vi "Process.vi"(0 "reference in":refnum<class "Battery.lvclass">, 5 "error in":errorcluster) -> (14 "reference out":refnum<class "Battery.lvclass">, 19 "error out":errorcluster)   [LabVIEW 2023, in "Battery.lvclass"]
uses:
  Battery.lvclass
  Model Parameters.ctl
  Simulation Parameters.ctl
  builds/PowerModuleInterface/PowerModuleInterface.lvlibp/Classes/PowerModule_interface/PowerModuleInterface.lvclass
  Battery.lvclass/Battery.ctl
  <vilib>/Utility/SystemLogging/NI_SystemLogging.lvlib
  <userlib>/_OpenG.lib/time/time.llb/openg_time.lvlib
panel:
  out "error info":errorcluster
  in  "Battery Tab Control":enum32{"MODEL", "SIMULATION", "PARAM"}(tab)
  out "SOC OCV Curve":cluster{"[0]":dbl, "[1]":dbl}[](graph)
  out "State of Charge %":dbl(slide)=100.0 caption="State of Charge (%)" scale=0.0..100.0 scale format="%.2g"
  out "Terminal Voltage (V)":dbl format="%#.3g"
  out "Battery Simulation":dbl[][](graph)
  out "Running Status Log":i32(listbox) caption="TEST SERVER LOG"
  out "Temperature (C)":dbl=25.0 format="%.2g"
  in  "Simulation Parameters":T1={"num_rc_pairs"=1, "R0"=0.0015, "R1"=0.001, "C1"=2500.0, "R2"=0.0008, "C2"=40000.0, " nominal_capacity_Ah"=5.0, "upper_voltage_cutoff"=4.2, "lower_voltage_cutoff"=3.0} {"lower_voltage_cutoff" format="%#_13g"; "upper_voltage_cutoff" format="%#_13g"; "nominal_capacity_Ah" format="%#_13g"; "C2" format="%#_13g"; "R2" format="%#_13g"; "C1" format="%#_13g"; "R1" format="%#_13g"; "R0" format="%#_13g"}
  in  "Model Parameters":T2={"chemistry"="Chen2020", "model_type"="SPMe"}
  out "Last Command":string
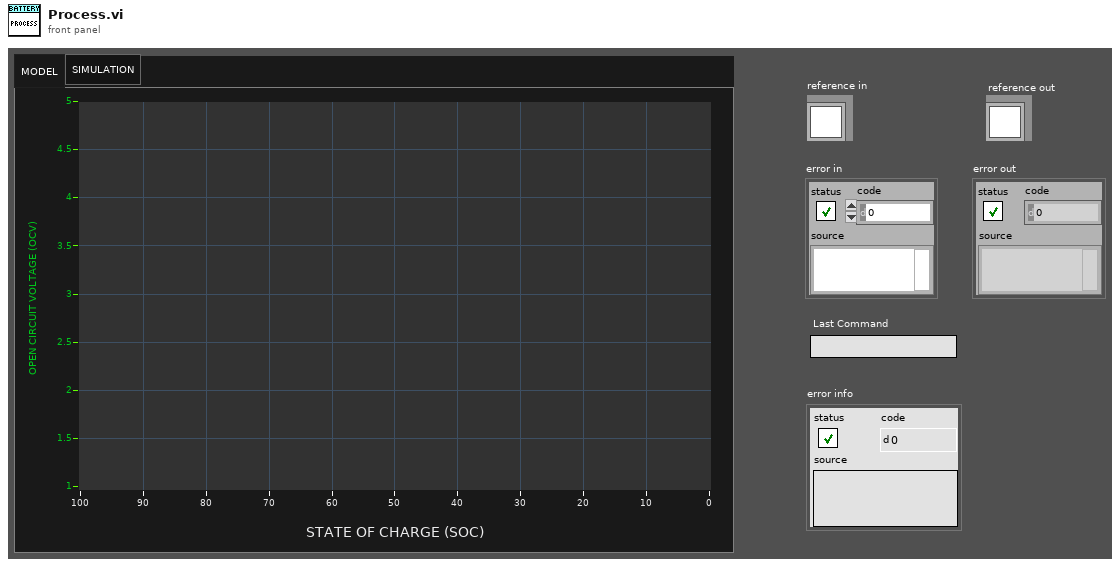
[diagram p1: front panel]
types:
  T1 = typedef "Battery.lvclass/Simulation Parameters.ctl" = cluster{"num_rc_pairs":i32, "R0":dbl, "R1":dbl, "C1":dbl, "R2":dbl, "C2":dbl, " nominal_capacity_Ah":dbl, "upper_voltage_cutoff":dbl, "lower_voltage_cutoff":dbl}
  T2 = typedef "Battery.lvclass/Model Parameters.ctl" = cluster{"chemistry":string, "model_type":string}
  T3 = cluster{"Core":cluster{"Timeout":i32, "Events":cluster{"EventsToProcess":refnum<event-registration>}, "EventFromProcess":refnum<user-event>, "ProcessSyncQueue":refnum<queue>, "QueueFromProcess":refnum<queue>, "Command":string, "Data":variant}}
  T4 = enum32{"Invalid", "Standard", "Closed", "Hidden", "Minimized", "Maximized"}
  T5 = cluster{"EventsToProcess":refnum<event-registration>}
  T6 = typedef "Battery.lvclass/ObjectAttributes.ctl" = cluster{"Python module":path, "Python Session":refnum<k35>, "PybammWrapper":refnum<k38>, "model loaded":bool, "simulation loaded":bool, "simulation enabled":bool, "SOC OCV Curve":dbl[][], "Open Circuit Voltage (V)":dbl, "State of Charge (%)":dbl, "# Cells in Series":u16, "# Cells in Parallel":u16, "Model Parameters":T2, "Simulation Parameters":T1, "Power Module":refnum<class "PowerModuleInterface.lvclass">}
  T7 = typedef "PowerModuleInterface.lvlibp/PowerModuleInterface.lvclass/Measurements.ctl" = cluster{"measured voltage (V)":dbl, "measured current (A)":dbl, "setpoint voltage (V)":dbl, "setpoint current (A)":dbl, "timestamp":dbl}
  T8 = cluster{"SOC OCV Curve[0]":dbl, "SOC OCV Curve[1]":dbl}
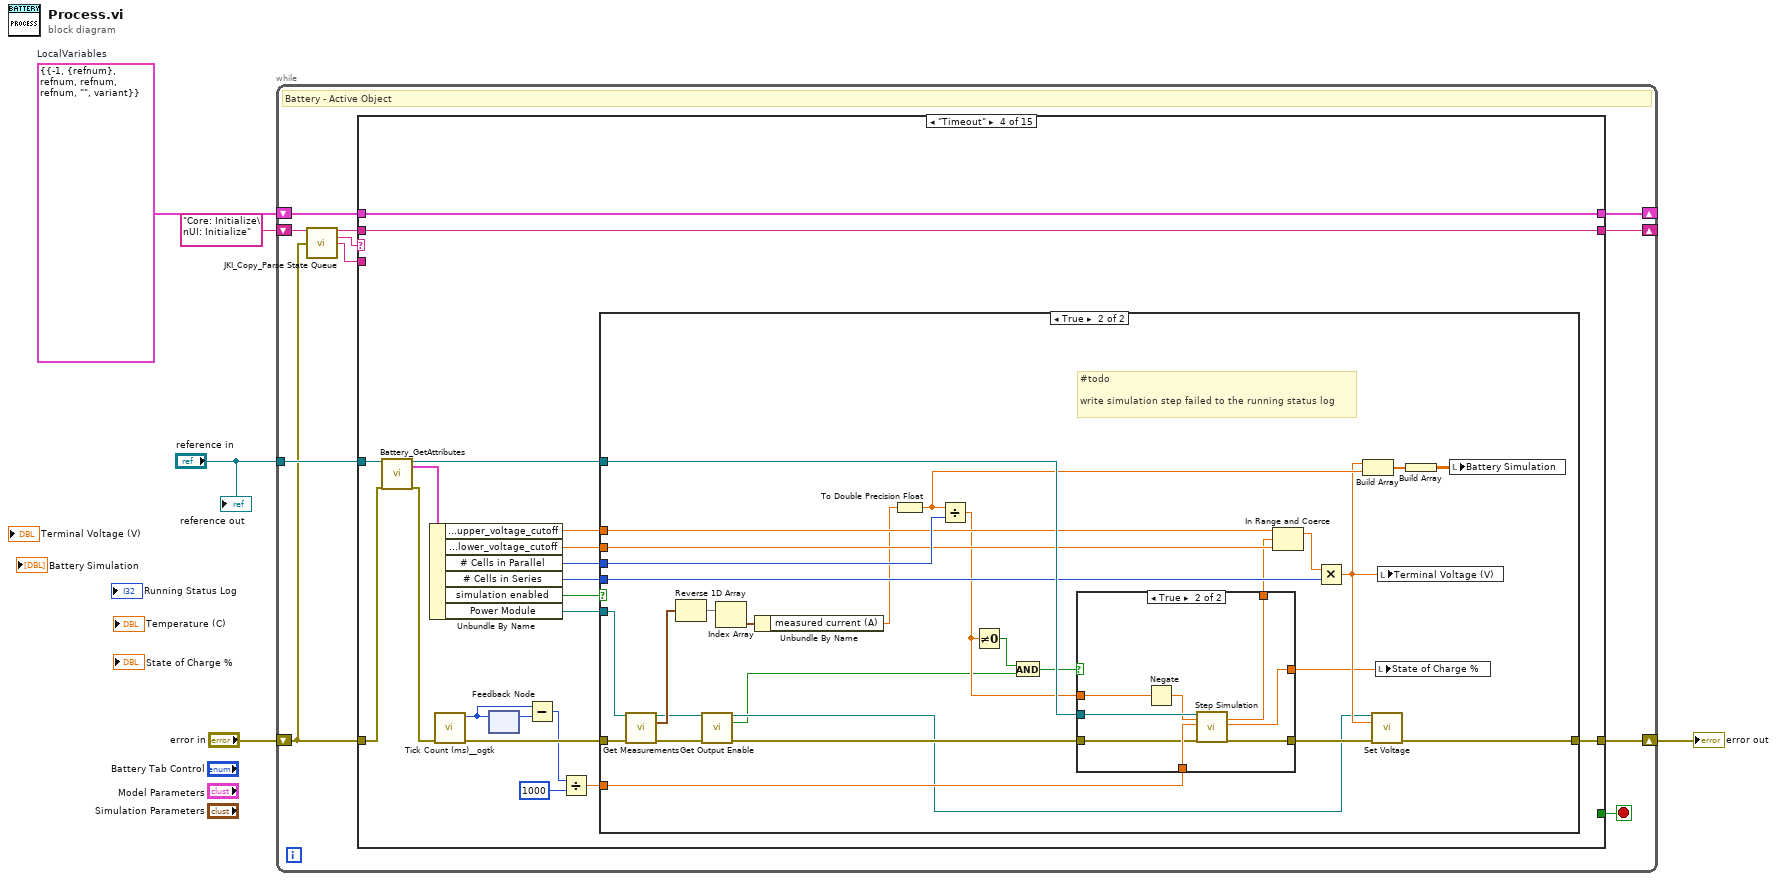
[diagram p0: block diagram]
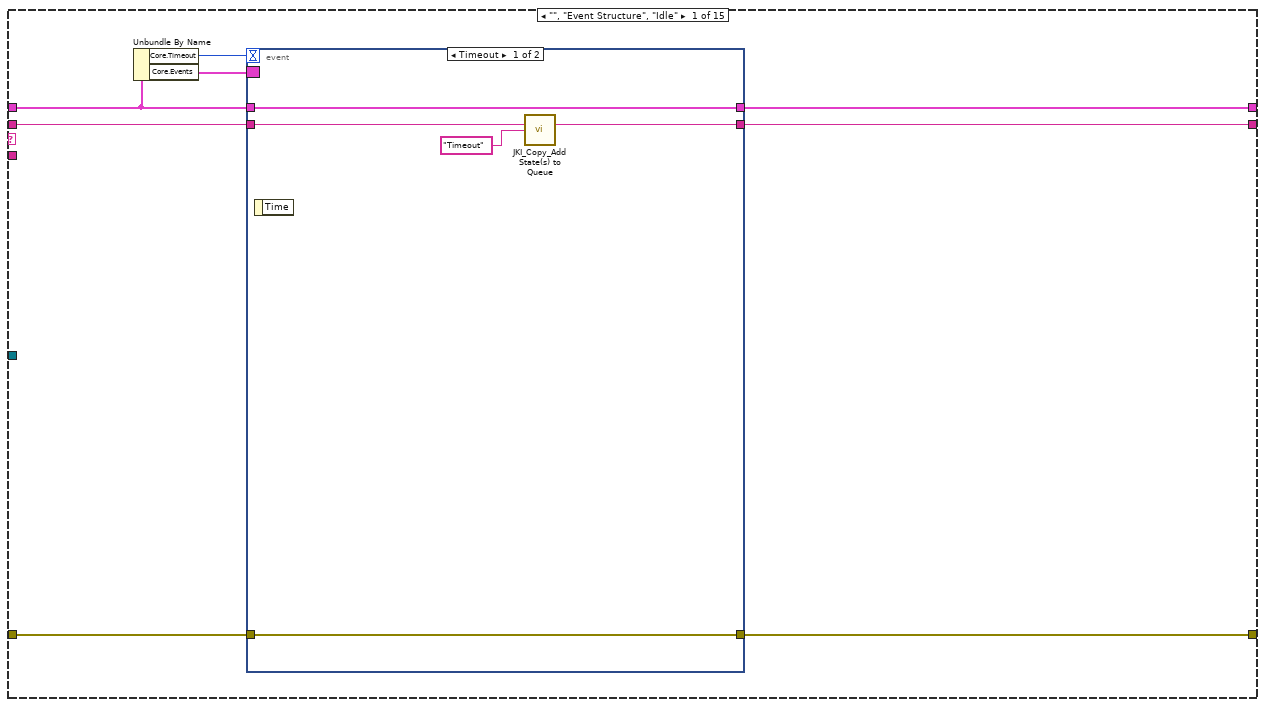
[diagram p2: hidden frame]
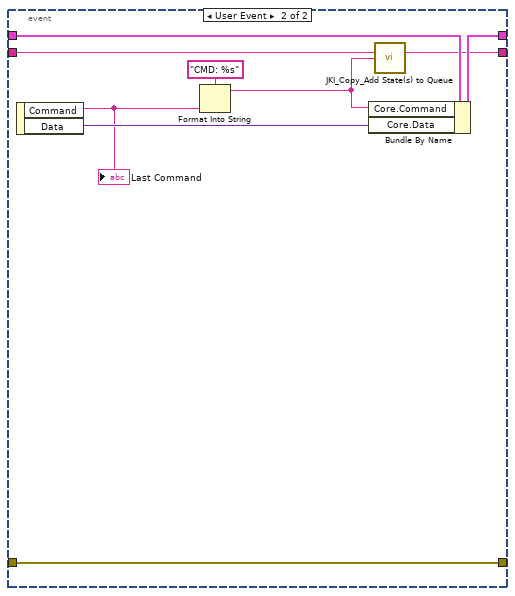
[diagram p3: hidden frame]
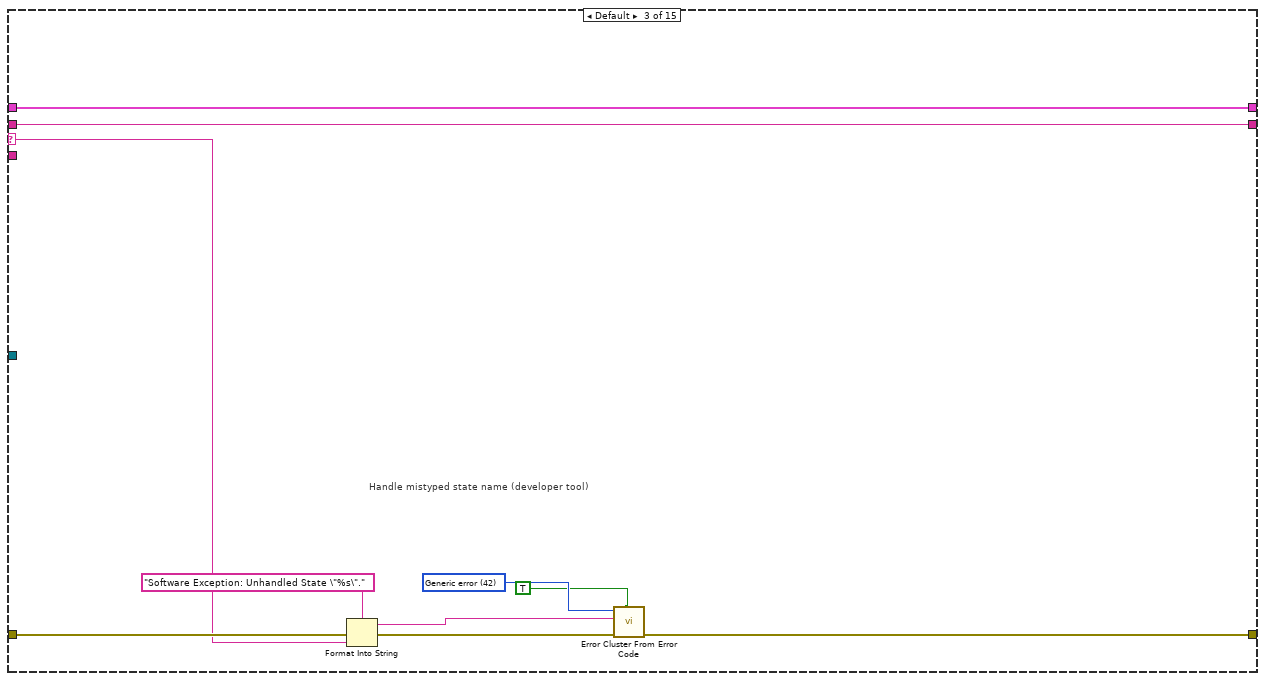
[diagram p5: hidden frame]
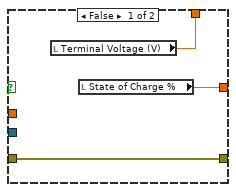
[diagram p7: hidden frame]
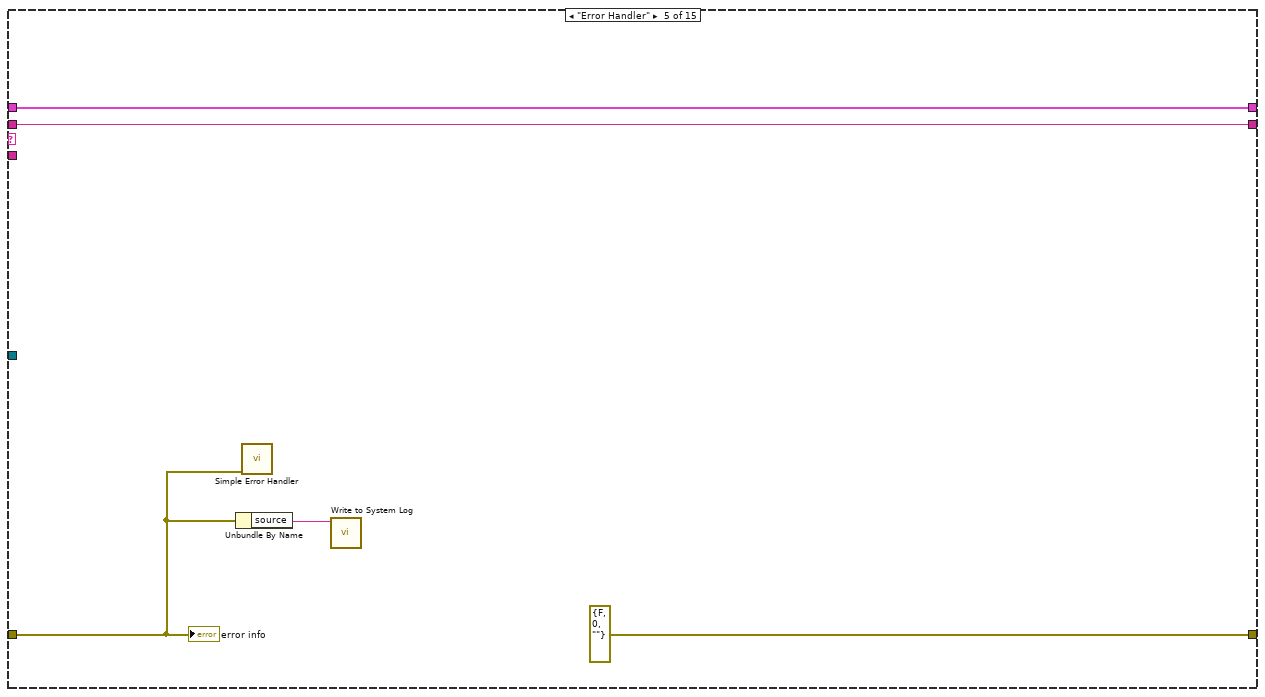
[diagram p8: hidden frame]
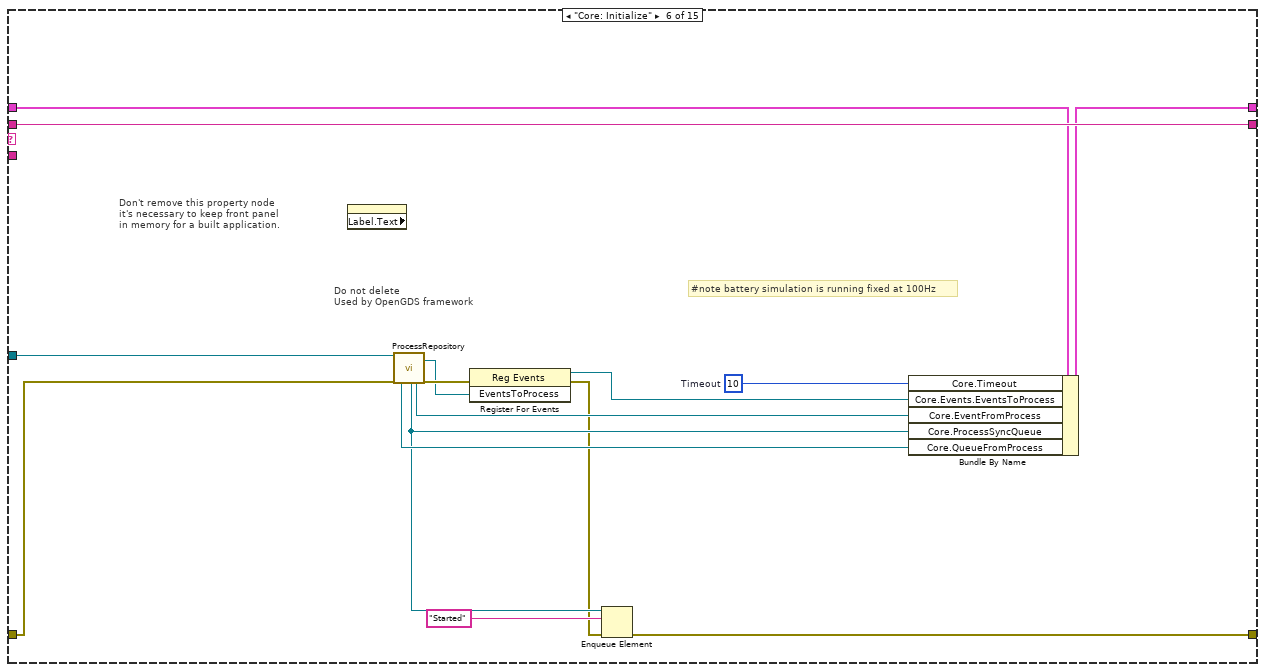
[diagram p9: hidden frame]
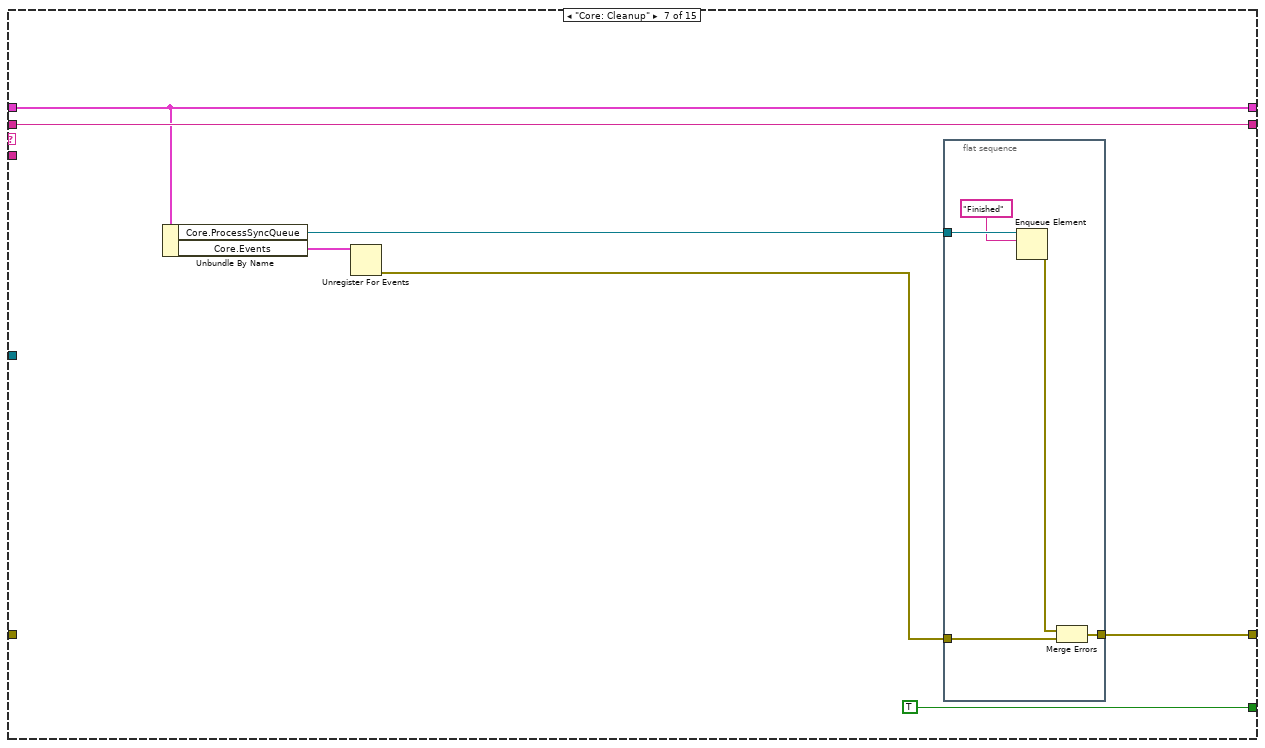
[diagram p10: hidden frame]
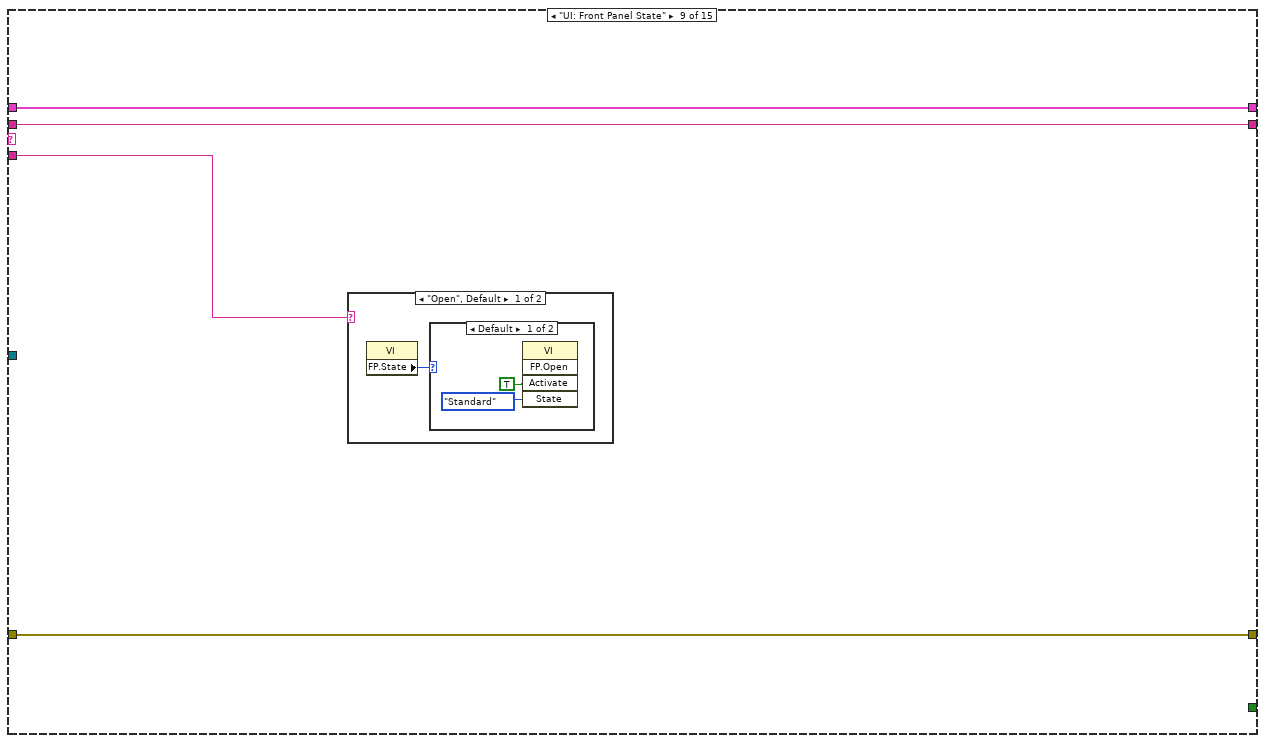
[diagram p12: hidden frame]
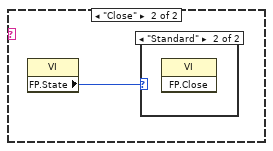
[diagram p14: hidden frame]
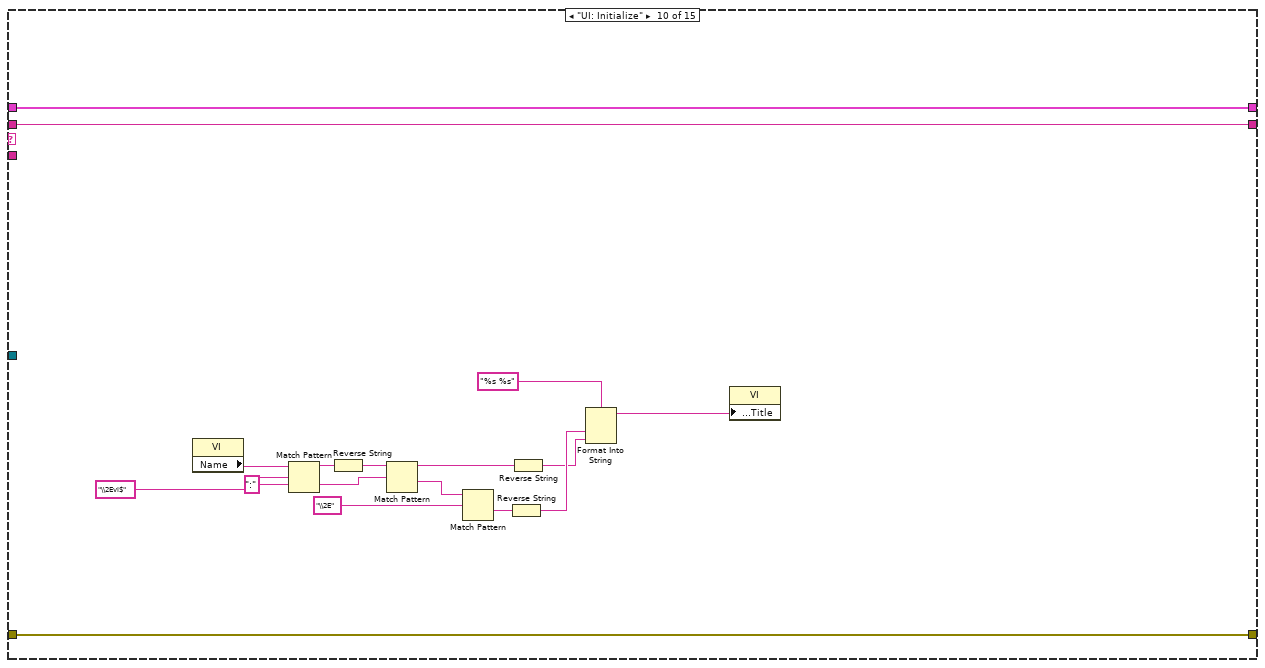
[diagram p16: hidden frame]
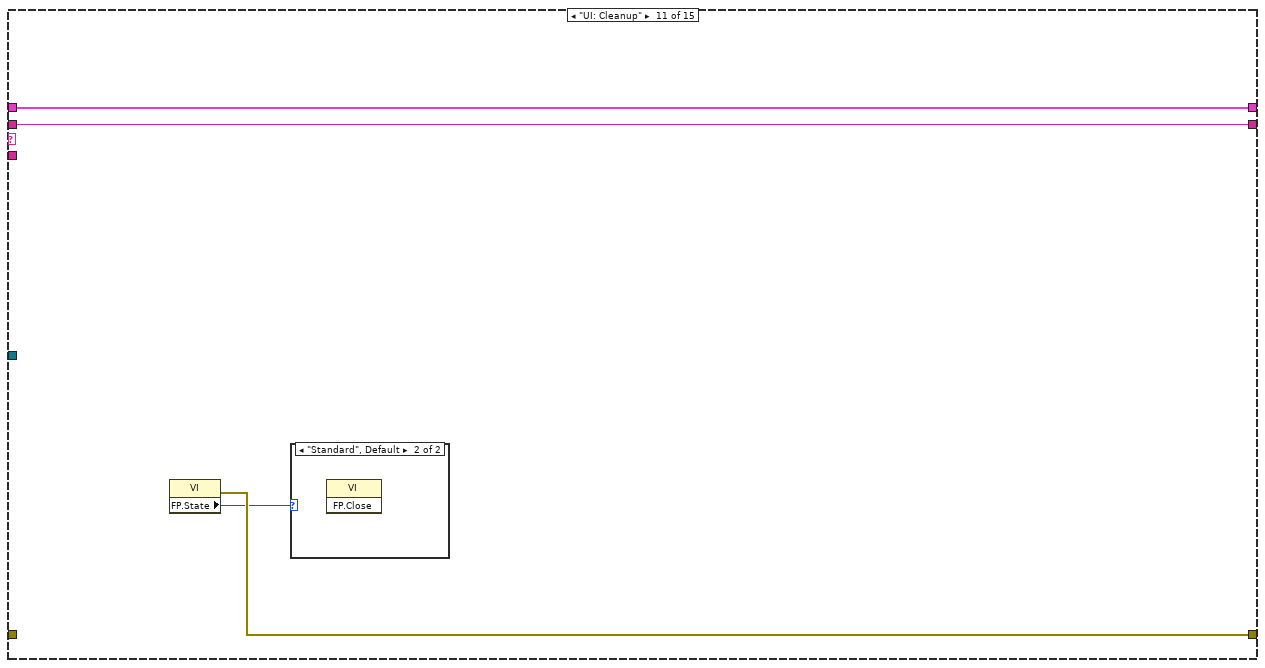
[diagram p17: hidden frame]
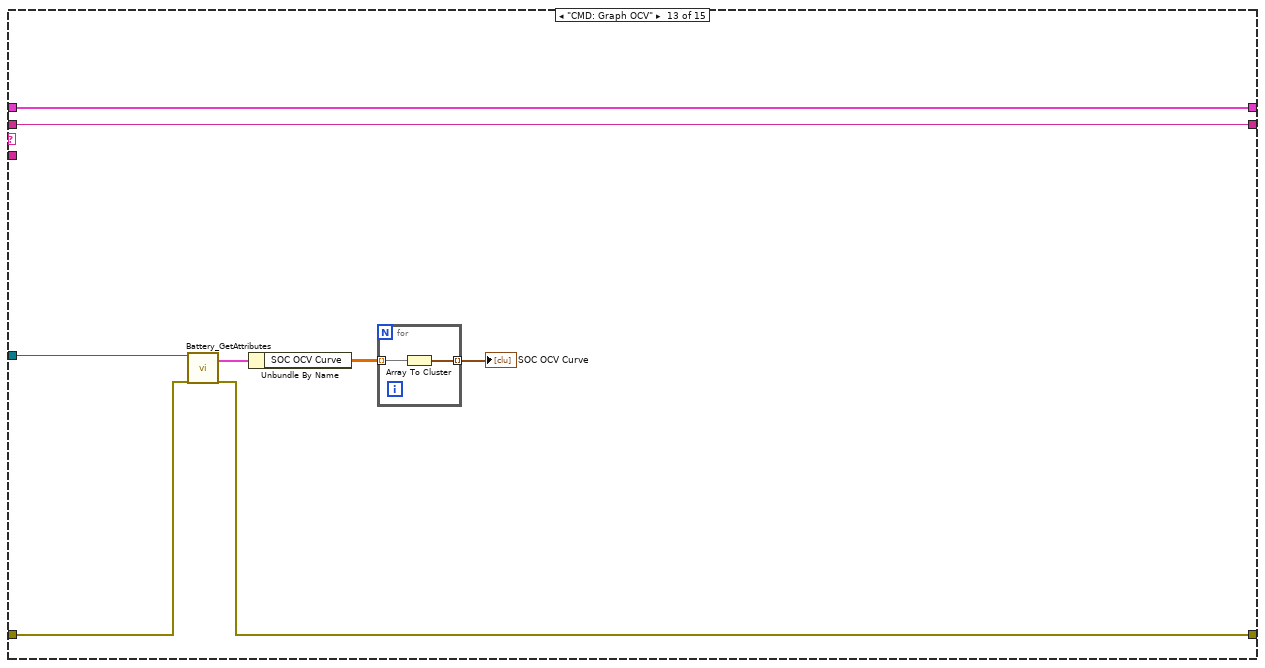
[diagram p20: hidden frame]
diagram:
  w5 = T3 {"Core"={"Timeout"=-1, "Events"={"EventsToProcess"=refnum}, "EventFromProcess"=refnum, "ProcessSyncQueue"=refnum, "QueueFromProcess"=refnum, "Command"="", "Data"=variant}}  # LocalVariables
  n1 = while {
    shift-right: [w16] -> w4
    shift-left: "error in" -> [w6]
    shift-right: [w13] -> _
    shift-left: "Core: Initialize\nUI: Initialize" ("States Out") -> [w10]
    shift-right: [w15] -> _
    shift-left: w5 -> [w14]
    tunnel: "reference in" -> [w11]
    stop <- w12 stop-if-true
    # "Battery - Active Object"
    n2 = call <vilib>:"JKI_Copy_Parse State Queue.vi"("State Queue"=w10, "Error In (no error)"=w6) -> ("Remaining States"=w9:string, "Current State"=w7:string, "Arguments"=w8:string)  [unwired: 11 in]
    n3 = case shown="\"Timeout\"" w7 {
      selector: w7 -> [_ _ w42 _ _ _ _ _ _ _ _ _ _ _ _]
      tunnel: w6 -> [w18 w41 w44 w61 w113 w118 _ w147 w148 w171 _ w178 w183 w191 w198]
      tunnel: [w19 w41 w43 w70 errorcluster {"status"=FALSE, "code"=0, "source"=""} ("error constant") w132 w135 w147 w148 w171 w173 w178 w182 w191 w198] -> w16
      tunnel: [w24 w40 w51 w52 w117 w130 w136 w146 w150 w169 w174 w177 w186 w190 w197] -> w15
      tunnel: w14 -> [w20 w40 w51 w52 w117 w129 w136 w146 w150 w169 w174 w177 w186 w190 w197]
      tunnel: w9 -> [w22 w39 w50 w71 w115 w131 w139 w145 w151 w170 w175 w176 w185 _ w195]
      tunnel: w8 -> [_ _ _ _ _ _ _ _ w149 _ _ _ _ _ _]
      tunnel: [w21 w39 w50 w71 w115 w131 w139 w145 w151 w170 w175 w176 w185 "UI: Cleanup\nCore: Cleanup" ("State(s) at Back (\"\")") w193] -> w13
      tunnel: [_ _ _ _ _ _ TRUE _ _ _ _ _ _ _ _] -> w12
      tunnel: w11 -> [_ _ _ w63 _ w119 _ _ _ _ _ _ w184 _ _]
      frame "", "Event Structure", "Idle" {
        n4 = Unbundle By Name(w20) -> ("Core.Timeout"=w17:i32, "Core.Events"=w23:T5)
        n5 = event shown="[0] Timeout" {
          selector: w23 -> [_ _]
          dyn-events: _ -> [_ _]
          timeout: w17 -> [_ _]
          tunnel: w20 -> [w29 w35]
          tunnel: [w29 w38] -> w24
          tunnel: [w26 w30] -> w21
          tunnel: w22 -> [w27 w31]
          tunnel: [w28 w36] -> w19
          tunnel: w18 -> [w28 w36]
          event Timeout {
            n6 = event-data() -> ()  [unwired: 1 in, 1 out]
            n7 = call <vilib>:"JKI_Copy_Add State(s) to Queue.vi"("State(s) in (\"\")"=w27, "State(s) at Back (\"\")"="Timeout" ("State(s) at Back (\"\")")) -> ("States Out"=w26:string)  [unwired: 13 in]
          }
          event User Event {
            n8 = event-data() -> ("Command"=w33:string, "Data"=w37:variant)  [unwired: 1 in]
            "Last Command" <- w33
            n9 = Format Into String(format string="CMD: %s", w33) -> (resulting string=w32:string)  [unwired: 2 in, 1 out]
            n10 = Bundle By Name(cluster=w35, "Core.Command"=w32, "Core.Data"=w37) -> (w38:T3)
            n11 = call <vilib>:"JKI_Copy_Add State(s) to Queue.vi"("State(s) in (\"\")"=w31, "State(s) at Back (\"\")"=w32) -> ("States Out"=w30:string)  [unwired: 13 in]
          }
        }
      }
      frame "---------- Core ----------" {
      }
      frame Default {
        w48 = 42 items=["No error", "Argument error", "Memory is full", "Out of zone", "End of file", "File already open", "Generic file I/O error", "File not found", "File permission error", "Disk is full", "Duplicate path", "Too many files open", "System feature not enabled", "Resource file not found", "Cannot add resource", "Resource not found", "Image not found", "Image memory error", "Pen does not exist", "Config type invalid", "Config token not found", "Config parse error", "Config memory error", "Bad external code format", "Bad external code offset", "External code not present", "Null window", "Destroy window error", "Null menu", "Print aborted", "Bad print record", "Print driver error", "Windows error during printing", "Memory error during printing", "Print dialog error", "Generic print error", "Invalid device refnum", "Device not found", "Device parameter error", "Device unit error", "Cannot open device", "Device call aborted", "Generic error", "Cancelled by user", "Object ID too low", "Object ID too high", "Object not in heap", "Unknown heap", "Unknown object (invalid DefProc)", "Unknown object (DefProc not in table)", "Message out of range", "Invalid (null) method", "Unknown message", "Manager call not supported", "Bad address", "Network operation in progress", "Network operation timed out", "Connection is busy", "Network attribute not supported", "Network error", "Address in use", "System out of memory", "Connection aborted", "Connection refused", "Not connected", "Already connected", "Connection closed", "Initialization error (interapplication manager)", "Bad occurrence", "Wait on unbound occurrence handler", "Occurrence queue overflow", "Datalog type conflict", "Unused", "Unrecognized type (interapplication manager)", "Memory corrupt", "Failed to make temporary DLL", "Old CIN version", "Drag socket not found", "Failed to load drop-object", "Failed to register OLE object", "Failed to release OLE object", "Format specifier type mismatch", "Unknown format specifier", "Too few format specifiers", "Too many format specifiers", "Scan failed", "Newer CIN version", "Error converting to variant", "Runtime menu error", "Password tampered", "Variant attribute not found", "Incompatible variant data type", "Event data is not available", "Event Store is not present", "Occurrence is not found", "Event Queue is not created", "Event info is not available", "Refnum passed is NULL", "Error retrieving Class GUID", "Error retrieving CoClass GUID", "Error retrieving TypeLib GUID.", "Bad built application magic bytes.", "Specific driver is different from the specific driver associated with the Logical Name.", "There is no session opened to the class driver.", "Max Error", "MAX - Error with config objects", "MAX - Error loading configuration", "MAX - Group not supported"]
        # "Handle mistyped state name (developer tool)"
        n12 = Format Into String(format string="Software Exception: Unhandled State \"%s\"." ("message"), error in=w44, w42) -> (resulting string=w47:string, error out=w46:errorcluster)  [unwired: 1 in]
        n13 = call <vilib>:"Error Cluster From Error Code.vi"("show call chain? (False)"=TRUE, "error in (no error)"=w46, "error message (\"\")"=w47, "error code (0)"=w48) -> ("error out"=w43:errorcluster)  [unwired: 5 in]
      }
      frame "Timeout" {
        n14 = call "Battery_GetAttributes.vi"("reference in"=w63, "Error In"=w61) -> ("reference out"=w62:refnum<class "Battery.lvclass">, "Data"=w59:T6, "Error Out"=w60:errorcluster)  [unwired: 14 in, 1 out]
        n15 = Unbundle By Name(w59) -> ("Simulation Parameters.upper_voltage_cutoff"=w53:dbl, "Simulation Parameters.lower_voltage_cutoff"=w54:dbl, "# Cells in Parallel"=w58:u16, "# Cells in Series"=w57:u16, "simulation enabled"=w56:bool, "Power Module"=w55:refnum<class "PowerModuleInterface.lvclass">)
        n16 = call <userlib>:"Tick Count (ms)__ogtk.vi"("error in (no error)"=w60) -> ("error out"=w69:errorcluster, "millisecond timer value"=w68:u32)  [unwired: 9 in]
        n17 = feedback-in #1(w68) -> ()
        n18 = feedback #1() -> (w67:u32)  [unwired: 1 in]
        n19 = Subtract(x=w68, y=w67) -> (x-y=w66:u32)
        n20 = Divide(x=w66, y=u32 1000) -> (x/y=w64:dbl)
        n21 = case shown="True" w56 {
          tunnel: w69 -> [w72 w89]
          tunnel: [w72 w100] -> w70
          tunnel: w62 -> [_ w101]
          tunnel: w64 -> [_ w98]
          tunnel: w58 -> [_ w97]
          tunnel: w57 -> [_ w94]
          tunnel: w55 -> [_ w88]
          tunnel: w54 -> [_ w96]
          tunnel: w53 -> [_ w95]
          frame False {
          }
          frame True {
            # "#todo\n\nwrite simulation step failed to the running status log"
            n22 = call-dynamic "Get Measurements.vi"("object in"=w88, "Error In"=w89) -> ("object out"=w77:refnum<class "PowerModuleInterface.lvclass">, "measurements"=w86:T7[], "Error Out"=w79:errorcluster)  [unwired: 11 in]
            n23 = Reverse 1D Array(array=w86) -> (reversed array=w85:T7[])
            n24 = call-dynamic "Get Output Enable.vi"("object in"=w77, "Error In"=w79) -> ("object out"=w76:refnum<class "PowerModuleInterface.lvclass">, "output"=w75:bool, "Error Out"=w78:errorcluster)  [unwired: 11 in]
            n25 = Index Array(array=w85) -> (element=w87:T7)  [unwired: 1 in]
            n26 = Unbundle By Name(w87) -> ("measured current (A)"=w93:dbl)
            n27 = To Double Precision Float(number=w93) -> (double precision float=w92:dbl)
            n28 = Divide(x=w92, y=w97) -> (x/y=w80:dbl)
            n29 = Not Equal To 0?(x=w80) -> (x != 0?=w74:bool)
            n30 = And(x=w74, y=w75) -> (x .and. y?=w73:bool)
            n31 = case shown="True" w73 {
              tunnel: w101 -> [_ w112]
              tunnel: w98 -> [_ w111]
              tunnel: w80 -> [_ w109]
              tunnel: w78 -> [w104 w108]
              tunnel: [w103 w107] -> w84
              tunnel: [w102 w106] -> w83
              tunnel: [w104 w105] -> w81
              frame False {
                n32 = local read "Terminal Voltage (V)"() -> (w102:dbl)
                n33 = local read "State of Charge %"() -> (w103:dbl)
              }
              frame True {
                n34 = Negate(x=w109) -> (-x=w110:dbl)
                n35 = call-dynamic "Step Simulation.vi"("reference in"=w112, "current_A"=w110, "time_step_S"=w111, "Error In"=w108) -> ("open circuit voltage"=w106:dbl, "state of charge"=w107:dbl, "Error Out"=w105:errorcluster)  [unwired: 11 in, 2 out]
              }
            }
            n36 = In Range and Coerce(upper limit=w95, x=w83, lower limit=w96) -> (coerced(x)=w82:dbl)  [unwired: 1 out]
            n37 = Multiply(x=w82, y=w94) -> (x*y=w91:dbl)
            n38 = Build Array(w91, w92) -> (w99:dbl[])
            n39 = call-dynamic "Set Voltage.vi"("object in"=w76, "voltage (V)"=w91, "Error In"=w81) -> ("Error Out"=w100:errorcluster)  [unwired: 11 in, 1 out]
            n40 = local write "State of Charge %"(w84) -> ()
            n41 = local write "Terminal Voltage (V)"(w91) -> ()
            n42 = Build Array(w99) -> (w90:dbl[][])
            n43 = local write "Battery Simulation"(w90) -> ()
          }
        }
      }
      frame "Error Handler" {
        n44 = Unbundle By Name(w113) -> ("source"=w114:string)
        n45 = call <vilib>:"Simple Error Handler.vi"("error in (no error)"=w113) -> ()  [unwired: 4 in, 5 out]
        n46 = call <vilib>:"Write to System Log.vi"("message"=w114) -> ()  [unwired: 10 in, 1 out]
        "error info" <- w113
      }
      frame "Core: Initialize" {
        w120 = 10  # Timeout
        # "#note battery simulation is running fixed at 100Hz"
        # "Do not delete\nUsed by OpenGDS framework"
        # "Don't remove this property node\nit's necessary to keep front panel\nin memory for a built application."
        # "Template created by VI Technologies"
        n47 = property on="reference in" class="LVClassControl (strict)" props=["Label", "Text"]() -> ()  [unwired: 2 in, 3 out]
        n48 = call "ProcessRepository.vi"("reference in"=w119, "Error In"=w118) -> ("QueueFromProcess"=w124:refnum<queue>, "ProcessSyncQueue"=w122:refnum<queue>, "EventFromProcess"=w125:refnum<user-event>, "EventsToProcess"=w127:refnum<user-event>, "Error Out"=w128:errorcluster)  [unwired: 10 in, 3 out]
        n49 = register-events(error in=w128, w127) -> (reference out=w126:refnum<event-registration>, error out=w121:errorcluster)  [unwired: 1 in]
        n50 = Enqueue Element(queue=w122, element="Started", error in (no error)=w121) -> (error out=w132:errorcluster)  [unwired: 1 in, 2 out]
        n51 = Bundle By Name(cluster=w129, "Core.Timeout"=w120, "Core.Events.EventsToProcess"=w126, "Core.EventFromProcess"=w125, "Core.ProcessSyncQueue"=w122, "Core.QueueFromProcess"=w124) -> (w130:T3)
      }
      frame "Core: Cleanup" {
        n52 = Unbundle By Name(w136) -> ("Core.ProcessSyncQueue"=w137:refnum<queue>, "Core.Events"=w134:T5)
        n53 = Unregister For Events(event registration refnum=w134) -> (error out=w133:errorcluster)  [unwired: 1 in]
        n54 = flat-sequence {
          tunnel: [w143] -> w135
          tunnel: w137 -> [w142]
          tunnel: w133 -> [w141]
          frame #0 {
            n55 = Enqueue Element(queue=w142, element="Finished") -> (error out=w144:errorcluster)  [unwired: 2 in, 2 out]
            n56 = Merge Errors(w144, w141) -> (w143:errorcluster)
          }
        }
      }
      frame "---------- UI ----------" {
      }
      frame "UI: Front Panel State" {
        n57 = case shown="\"Open\", Default" w149 {
          frame "Open", Default {
            n58 = property class="VI"() -> ("FP.State"=w152:T4)  [unwired: 2 in, 2 out]
            n59 = case shown="Default" w152 {
              frame Default {
                n60 = invoke class="VI" method="FP.Open"("Activate"=TRUE, "State"=T4."Standard") -> ()  [unwired: 3 in, 5 out]
              }
              frame "Standard" {
              }
            }
          }
          frame "Close" {
            n61 = property class="VI"() -> ("FP.State"=w155:T4)  [unwired: 2 in, 2 out]
            n62 = case shown="\"Standard\"" w155 {
              frame Default {
              }
              frame "Standard" {
                n63 = invoke class="VI" method="FP.Close"() -> ()  [unwired: 3 in, 3 out]
              }
            }
          }
        }
      }
      frame "UI: Initialize" {
        n64 = property class="VI"() -> ("Name"=w168:string)  [unwired: 2 in, 2 out]
        n65 = Match Pattern(string=w168, regular expression="\\2Evi$") -> (before substring=w166:string)  [unwired: 1 in, 3 out]
        n66 = Reverse String(1:w166) -> (0:w165:string)
        n67 = Match Pattern(string=w165, regular expression=":") -> (before substring=w163:string, after substring=w162:string)  [unwired: 1 in, 2 out]
        n68 = Match Pattern(string=w162, regular expression="\\2E") -> (after substring=w160:string)  [unwired: 1 in, 3 out]
        n69 = Reverse String(1:w160) -> (0:w159:string)
        n70 = Reverse String(1:w163) -> (0:w158:string)
        n71 = Format Into String(format string="%s %s", w159, w158) -> (resulting string=w157:string)  [unwired: 2 in, 1 out]
        n72 = property class="VI"("Front Panel.Title"=w157) -> ()  [unwired: 2 in, 2 out]
      }
      frame "UI: Cleanup" {
        n73 = property class="VI"() -> (error out=w173:errorcluster, "FP.State"=w172:T4)  [unwired: 2 in, 1 out]
        n74 = case shown="\"Standard\", Default" w172 {
          frame "Closed" {
          }
          frame "Standard", Default {
            n75 = invoke class="VI" method="FP.Close"() -> ()  [unwired: 3 in, 3 out]
          }
        }
      }
      frame "-------- CMD --------" {
      }
      frame "CMD: Graph OCV" {
        n76 = call "Battery_GetAttributes.vi"("reference in"=w184, "Error In"=w183) -> ("Data"=w181:T6, "Error Out"=w182:errorcluster)  [unwired: 14 in, 2 out]
        n77 = Unbundle By Name(w181) -> ("SOC OCV Curve"=w179:dbl[][])
        n78 = for {
          tunnel: w179 -> [w188] mode=indexing
          tunnel: [w187] -> w180 mode=indexing
          n79 = Array To Cluster(array=w188) -> (cluster=w187:T8)
        }
        "SOC OCV Curve" <- w180
      }
      frame "CMD: Exit" {
      }
      frame "CMD: Front Panel State" {
        n80 = Format Into String(format string="UI: Front Panel State>>%s" ("string"), "Open" ("input 1")) -> (resulting string=w194:string)  [unwired: 2 in, 1 out]
        n81 = call <vilib>:"JKI_Copy_Add State(s) to Queue.vi"("State(s) in (\"\")"=w195, "State(s) at Back (\"\")"=w194) -> ("States Out"=w193:string)  [unwired: 13 in]
      }
    }
  }
  "error out" <- w4
  "reference out" <- "reference in"
